vi "FGGA TCP Packet_v2.vi"(0 "ID":string, 1 "dummy2":string="0", 5 "Version":string, 7 "utc_time":u32, 9 "dummy1":string="0", 11 "Flight Number":string, 12 "Data Array":string[](array[string]), 13 "ch4_dry":string, 14 "co2_dry":string) -> (8 "TCP Binary Packet":string)   [LabVIEW 2014]
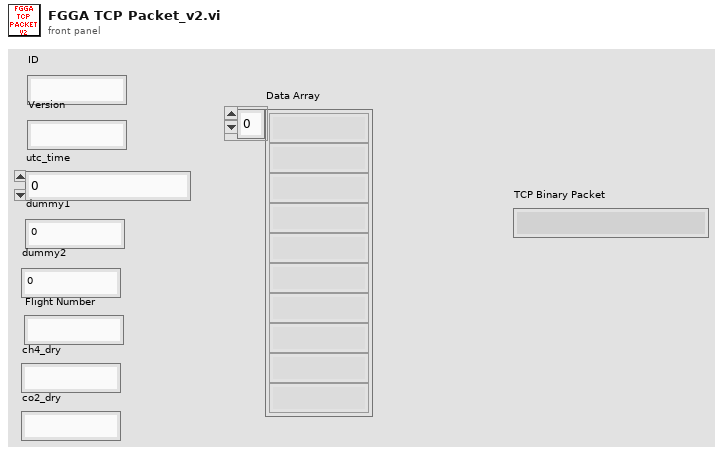
[diagram p1: front panel]
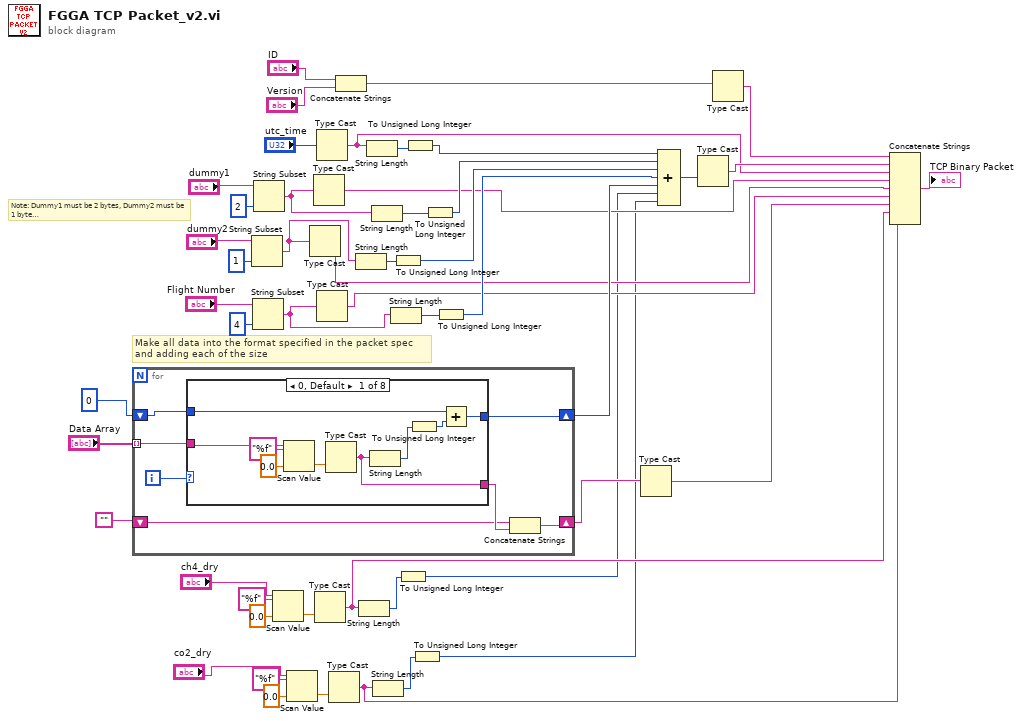
[diagram p0: block diagram]
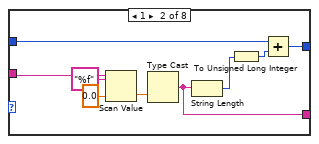
[diagram p2: hidden frame]
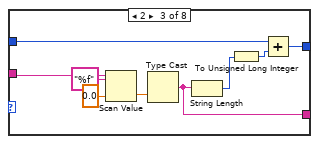
[diagram p3: hidden frame]
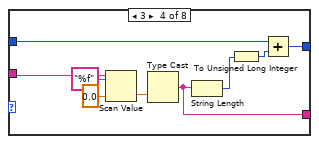
[diagram p4: hidden frame]
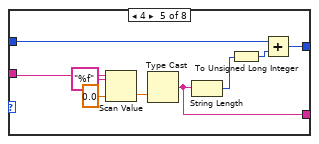
[diagram p5: hidden frame]
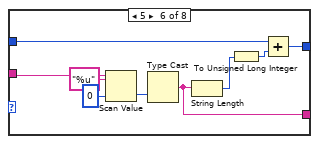
[diagram p6: hidden frame]
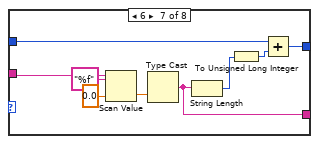
[diagram p7: hidden frame]
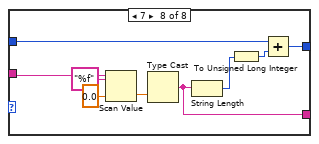
[diagram p8: hidden frame]
diagram:
  # "Note: Dummy1 must be 2 bytes, Dummy2 must be 1 byte\nin order to make the Flight number to start from byte 20"
  # "Make all data into the format specified in the packet spec\nand adding each of the size"
  n1 = for {
    tunnel: "Data Array" -> [w55] mode=indexing
    shift-right: [w53] -> w31
    shift-left: u32 0 -> [w54]
    shift-right: [w52] -> w19
    shift-left: "" -> [w50]
    i -> [w56]
    n2 = case shown="0, Default" w56 {
      tunnel: w55 -> [w63 w72 w81 w90 w99 w108 w117 w126]
      tunnel: w54 -> [w61 w70 w79 w88 w97 w106 w115 w124]
      tunnel: [w58 w67 w76 w85 w94 w103 w112 w121] -> w53
      tunnel: [w57 w66 w75 w84 w93 w102 w111 w120] -> w51
      frame 0, Default {
        n3 = Scan Value(string=w63, format string="%f", default (0 dbl)=sgl 0.0 ("default (0 I32)")) -> (value=w65:sgl)  [unwired: 1 out]
        n4 = Type Cast(x=w65) -> (*(type *) &x=w57:string)  [unwired: 1 in]
        n5 = String Length(string=w57) -> (length=w60:i32)
        n6 = To Unsigned Long Integer(number=w60) -> (unsigned 32bit integer=w59:u32)
        n7 = Add(x=w61, y=w59) -> (x+y=w58:u32)
      }
      frame 1 {
        n8 = Scan Value(string=w72, format string="%f", default (0 dbl)=sgl 0.0 ("default (0 I32)")) -> (value=w74:sgl)  [unwired: 1 out]
        n9 = Type Cast(x=w74) -> (*(type *) &x=w66:string)  [unwired: 1 in]
        n10 = String Length(string=w66) -> (length=w69:i32)
        n11 = To Unsigned Long Integer(number=w69) -> (unsigned 32bit integer=w68:u32)
        n12 = Add(x=w70, y=w68) -> (x+y=w67:u32)
      }
      frame 2 {
        n13 = Scan Value(string=w81, format string="%f", default (0 dbl)=sgl 0.0 ("default (0 I32)")) -> (value=w83:sgl)  [unwired: 1 out]
        n14 = Type Cast(x=w83) -> (*(type *) &x=w75:string)  [unwired: 1 in]
        n15 = String Length(string=w75) -> (length=w78:i32)
        n16 = To Unsigned Long Integer(number=w78) -> (unsigned 32bit integer=w77:u32)
        n17 = Add(x=w79, y=w77) -> (x+y=w76:u32)
      }
      frame 3 {
        n18 = Scan Value(string=w90, format string="%f", default (0 dbl)=sgl 0.0 ("default (0 I32)")) -> (value=w92:sgl)  [unwired: 1 out]
        n19 = Type Cast(x=w92) -> (*(type *) &x=w84:string)  [unwired: 1 in]
        n20 = String Length(string=w84) -> (length=w87:i32)
        n21 = To Unsigned Long Integer(number=w87) -> (unsigned 32bit integer=w86:u32)
        n22 = Add(x=w88, y=w86) -> (x+y=w85:u32)
      }
      frame 4 {
        n23 = Scan Value(string=w99, format string="%f", default (0 dbl)=sgl 0.0 ("default (0 I32)")) -> (value=w101:sgl)  [unwired: 1 out]
        n24 = Type Cast(x=w101) -> (*(type *) &x=w93:string)  [unwired: 1 in]
        n25 = String Length(string=w93) -> (length=w96:i32)
        n26 = To Unsigned Long Integer(number=w96) -> (unsigned 32bit integer=w95:u32)
        n27 = Add(x=w97, y=w95) -> (x+y=w94:u32)
      }
      frame 5 {
        n28 = Scan Value(string=w108, format string="%u", default (0 dbl)=u16 0 ("default (0 I32)")) -> (value=w110:u16)  [unwired: 1 out]
        n29 = Type Cast(x=w110) -> (*(type *) &x=w102:string)  [unwired: 1 in]
        n30 = String Length(string=w102) -> (length=w105:i32)
        n31 = To Unsigned Long Integer(number=w105) -> (unsigned 32bit integer=w104:u32)
        n32 = Add(x=w106, y=w104) -> (x+y=w103:u32)
      }
      frame 6 {
        n33 = Scan Value(string=w117, format string="%f", default (0 dbl)=sgl 0.0 ("default (0 I32)")) -> (value=w119:sgl)  [unwired: 1 out]
        n34 = Type Cast(x=w119) -> (*(type *) &x=w111:string)  [unwired: 1 in]
        n35 = String Length(string=w111) -> (length=w114:i32)
        n36 = To Unsigned Long Integer(number=w114) -> (unsigned 32bit integer=w113:u32)
        n37 = Add(x=w115, y=w113) -> (x+y=w112:u32)
      }
      frame 7 {
        n38 = Scan Value(string=w126, format string="%f", default (0 dbl)=sgl 0.0 ("default (0 I32)")) -> (value=w128:sgl)  [unwired: 1 out]
        n39 = Type Cast(x=w128) -> (*(type *) &x=w120:string)  [unwired: 1 in]
        n40 = String Length(string=w120) -> (length=w123:i32)
        n41 = To Unsigned Long Integer(number=w123) -> (unsigned 32bit integer=w122:u32)
        n42 = Add(x=w124, y=w122) -> (x+y=w121:u32)
      }
    }
    n43 = Concatenate Strings(w50, w51) -> (w52:string)
  }
  n44 = String Subset(string="dummy2", length (rest)=1 ("length (rest)")) -> (substring=w16:string)  [unwired: 1 in]
  n45 = String Subset(string="Flight Number", length (rest)=4 ("length (rest)")) -> (substring=w23:string)  [unwired: 1 in]
  n46 = String Subset(string="dummy1", length (rest)=2 ("length (rest)")) -> (substring=w26:string)  [unwired: 1 in]
  n47 = Scan Value(string="ch4_dry", format string="%f", default (0 dbl)=sgl 0.0 ("default (0 I32)")) -> (value=w14:sgl)  [unwired: 1 out]
  n48 = Scan Value(string="co2_dry", format string="%f", default (0 dbl)=sgl 0.0 ("default (0 I32)")) -> (value=w7:sgl)  [unwired: 1 out]
  n49 = Type Cast(x=w16) -> (*(type *) &x=w15:string)  [unwired: 1 in]
  n50 = Type Cast(x=w26) -> (*(type *) &x=w25:string)  [unwired: 1 in]
  n51 = Type Cast(x=w14) -> (*(type *) &x=w9:string)  [unwired: 1 in]
  n52 = Type Cast(x="utc_time") -> (*(type *) &x=w27:string)  [unwired: 1 in]
  n53 = Type Cast(x=w23) -> (*(type *) &x=w24:string)  [unwired: 1 in]
  n54 = Type Cast(x=w7) -> (*(type *) &x=w1:string)  [unwired: 1 in]
  n55 = Concatenate Strings("ID", "Version") -> (w47:string)
  n56 = String Length(string=w16) -> (length=w39:i32)
  n57 = String Length(string=w9) -> (length=w11:i32)
  n58 = String Length(string=w27) -> (length=w46:i32)
  n59 = String Length(string=w26) -> (length=w42:i32)
  n60 = String Length(string=w1) -> (length=w4:i32)
  n61 = String Length(string=w23) -> (length=w36:i32)
  n62 = To Unsigned Long Integer(number=w39) -> (unsigned 32bit integer=w38:u32)
  n63 = To Unsigned Long Integer(number=w11) -> (unsigned 32bit integer=w8:u32)
  n64 = To Unsigned Long Integer(number=w46) -> (unsigned 32bit integer=w44:u32)
  n65 = To Unsigned Long Integer(number=w4) -> (unsigned 32bit integer=w2:u32)
  n66 = To Unsigned Long Integer(number=w42) -> (unsigned 32bit integer=w40:u32)
  n67 = To Unsigned Long Integer(number=w36) -> (unsigned 32bit integer=w34:u32)
  n68 = Type Cast(x=w19) -> (*(type *) &x=w22:string)  [unwired: 1 in]
  n69 = Compound Arithmetic op=ADD(w44, w40, w38, w34, w31, w8, w2) -> (w29:u32)
  n70 = Type Cast(x=w29) -> (*(type *) &x=w28:string)  [unwired: 1 in]
  n71 = Type Cast(x=w47) -> (*(type *) &x=w30:string)  [unwired: 1 in]
  n72 = Concatenate Strings(w30, w28, w27, w25, w15, w24, w22, w9, w1) -> (→"TCP Binary Packet":string)
